vi "Page Number Formatted string.vi"(0 "Page #":i32, 7 "Total page #":i32, 11 "Page # cluster":T1) -> (4 "Temporaty Cell":string, 8 "Page string":string, 15 "Final Cell":string)   [LabVIEW 2012]
doc: "Version 1.0\nDeveloped by Jean-Marc Simard\nCopyright © 2010, Exaprom Inc.\nAll rights reserved.\nLicense: BSD"
uses:
  Controls/Page number.ctl
panel:
  # "Y"
  # "X"
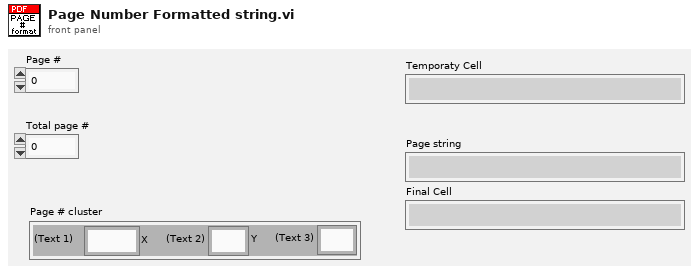
[diagram p1: front panel]
types:
  T1 = typedef "Page number.ctl" = cluster{"Text 1":string, "Text 2":string, "Text 3":string}
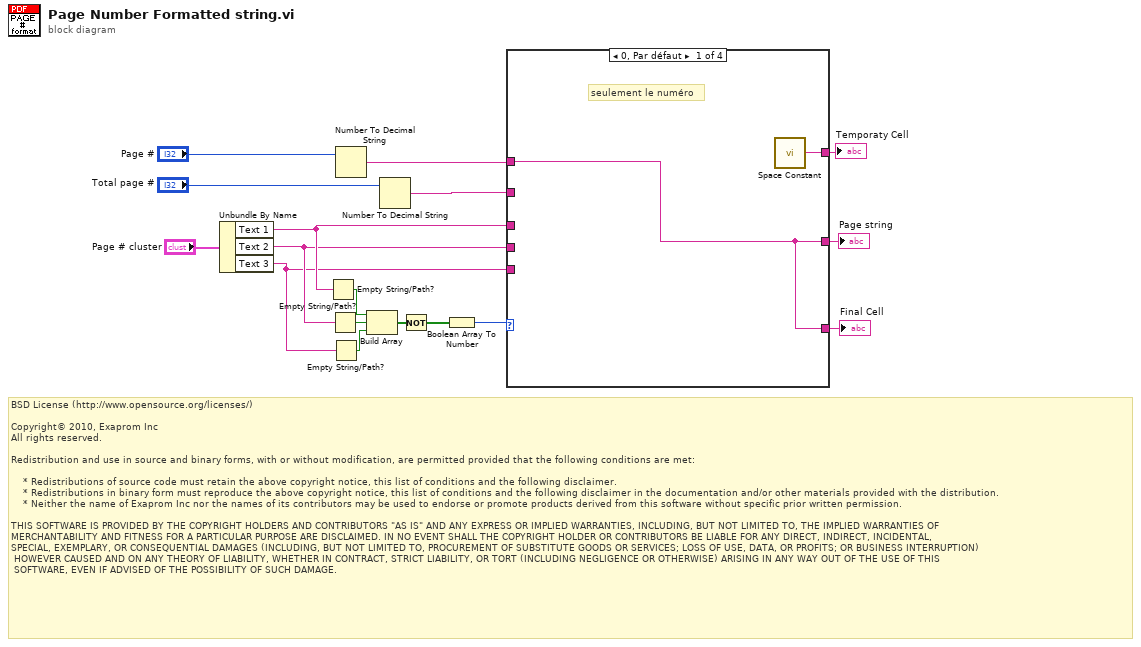
[diagram p0: block diagram]
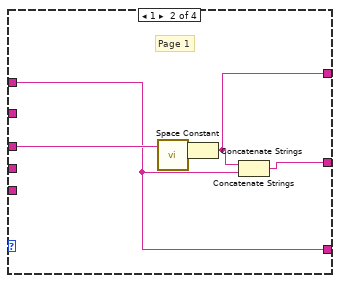
[diagram p2: hidden frame]
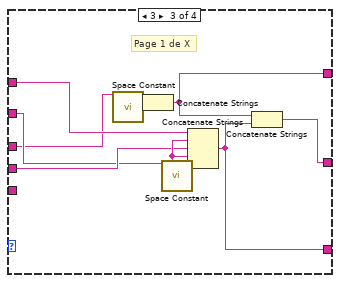
[diagram p3: hidden frame]
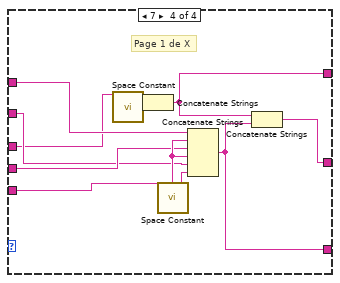
[diagram p4: hidden frame]
diagram:
  # "BSD License (http://www.opensource.org/licenses/)\n\nCopyright© 2010, Exaprom Inc\nAll rights reserved.\n\nRedistribution and use in source and binary forms, with or without modification, are permitted provided that the following conditions are met:\n\n    * Redistributions of source code must retain the above copyright notice, this list of conditions and the following disclaimer.\n    * Redistributions in binary form must reproduce the above copyright notice, this list of conditions and the following disclaimer in the documentation and/or other materials provided with the distribution.\n    * Neither the name of Exaprom Inc nor the names of its contributors may be used to endorse or promote products derived from this software without specific prior written permission.\n\nTHIS SOFTWARE IS PROVIDED BY THE COPYRIGHT HOLDERS AND CONTRIBUTORS \"AS IS\" AND ANY EXPRESS OR IMPLIED WARRANTIES, INCLUDING, BUT NOT LIMITED TO, THE IMPLIED WARRANTIES OF \nMERCHANTABILITY AND FITNESS FOR A PARTICULAR PURPOSE ARE DISCLAIMED. IN NO EVENT SHALL THE COPYRIGHT HOLDER OR CONTRIBUTORS BE LIABLE FOR ANY DIRECT, INDIRECT, INCIDENTAL,\nSPECIAL, EXEMPLARY, OR CONSEQUENTIAL DAMAGES (INCLUDING, BUT NOT LIMITED TO, PROCUREMENT OF SUBSTITUTE GOODS OR SERVICES; LOSS OF USE, DATA, OR PROFITS; OR BUSINESS INTERRUPTION)\n HOWEVER CAUSED AND ON ANY THEORY OF LIABILITY, WHETHER IN CONTRACT, STRICT LIABILITY, OR TORT (INCLUDING NEGLIGENCE OR OTHERWISE) ARISING IN ANY WAY OUT OF THE USE OF THIS\n SOFTWARE, EVEN IF ADVISED OF THE POSSIBILITY OF SUCH DAMAGE."
  n1 = Unbundle By Name("Page # cluster") -> ("Text 1"=w8:string, "Text 2"=w7:string, "Text 3"=w6:string)
  n2 = Empty String/Path?(string/path=w8) -> (empty?=w16:bool)
  n3 = Empty String/Path?(string/path=w7) -> (empty?=w15:bool)
  n4 = Empty String/Path?(string/path=w6) -> (empty?=w14:bool)
  n5 = Number To Decimal String(number="Page #") -> (decimal integer string=w4:string)  [unwired: 1 out]
  n6 = Build Array(w16, w15, w14) -> (w13:bool[])
  n7 = Number To Decimal String(number="Total page #") -> (decimal integer string=w9:string)  [unwired: 1 out]
  n8 = Not(x=w13) -> (.not. x?=w5:bool[])
  n9 = Boolean Array To Number(Boolean array=w5) -> (number=w12:u32)
  n10 = case shown="0, Par défaut" w12 {
    tunnel: w8 -> [_ w23 w28 w38]
    tunnel: w7 -> [_ _ w31 w41]
    tunnel: w6 -> [_ _ _ w34]
    tunnel: w4 -> [w19 w20 w32 w42]
    tunnel: w9 -> [_ _ w30 w40]
    tunnel: [w19 w22 w25 w35] -> w3
    tunnel: [w18 w21 w27 w37] -> w2
    tunnel: [w19 w20 w26 w36] -> w1
    frame 0, Default {
      # "seulement le numéro"
      n11 = call <vilib>:"Space Constant.vi"() -> ("String"=w18:string)
    }
    frame 1 {
      # "Page 1"
      n12 = call <vilib>:"Space Constant.vi"() -> ("String"=w24:string)
      n13 = Concatenate Strings(w23, w24) -> (w21:string)
      n14 = Concatenate Strings(w21, w20) -> (w22:string)
    }
    frame 3 {
      # "Page 1 de X"
      n15 = call <vilib>:"Space Constant.vi"() -> ("String"=w29:string)
      n16 = Concatenate Strings(w28, w29) -> (w27:string)
      n17 = call <vilib>:"Space Constant.vi"() -> ("String"=w33:string)
      n18 = Concatenate Strings(w32, w33, w31, w33, w30) -> (w26:string)
      n19 = Concatenate Strings(w27, w26) -> (w25:string)
    }
    frame 7 {
      # "Page 1 de X"
      n20 = call <vilib>:"Space Constant.vi"() -> ("String"=w39:string)
      n21 = Concatenate Strings(w38, w39) -> (w37:string)
      n22 = call <vilib>:"Space Constant.vi"() -> ("String"=w43:string)
      n23 = Concatenate Strings(w42, w43, w41, w43, w40, w34) -> (w36:string)
      n24 = Concatenate Strings(w37, w36) -> (w35:string)
    }
  }
  "Page string" <- w3
  "Temporaty Cell" <- w2
  "Final Cell" <- w1
